vi "set Komp changes.vi"(7 "init":bool, 8 "Fehler (Eingang, kein Fehler)":errorcluster, 9 "Changes":T1, 11 "TestKonfig (Eingang) (Eingang)":T3 {"TestKonfig Interferent"."Gasflasche MFC3" items=["----"=10000, "IAG NH3 3000"=0, "IAG NH3 200"=1, "IAG NH3 2000"=2, "IAG MG"=3, "IAG O2"=4]; "TestKonfig Interferent"."Gasflasche MFC2" items=["----"=10000, "IAG NH3 3000"=0, "IAG NH3 200"=1, "IAG NH3 2000"=2, "IAG MG"=3, "IAG O2"=4]; "TestKonfig Interferent"."Eingangs Konzentration MFC1" min=0.0; "TestKonfig Interferent"."Ausgangs Konzentration MFC1" min=0.0; "TestKonfig Interferent"."MFC2" items=["MFC 2", "MFC 3", "MFC 4", "MFC 5"]; "TestKonfig Interferent"."MFC3" items=["MFC 2", "MFC 3", "MFC 4", "MFC 5"]; "TestKonfig Interferent"."Ausgangs Konzentration MFC3" min=0.0; "TestKonfig Interferent"."Eingangs Konzentration MFC3" min=0.0; "TestKonfig Interferent"."Ausgangs Konzentration MFC2" min=0.0; "TestKonfig Interferent"."Eingangs Konzentration MFC2" min=0.0; "TestKonfig H2O"."HovaCAL Temperature" format="%.2f"; "TestKonfig H2O"."HovaCAL Flow Input Cluster"."HovaCAL Flow Input Cluster" format="%.2f"; "TestKonfig H2O"."Eingangs Konzentration:" min=0.0; "TestKonfig H2O"."zusätzliche Zeitdauer Erster Punkt" min=30 step=1 format="%#_5g"; "TestKonfig H2O"."Zeitdauer Stufen" format="%#_5g"; "TestKonfig H2O"."Max Fehler" format="%#_5g"; "TestKonfig H2O"."Anzahl Stufen" format="%#_5g"; "TestKonfig H2O"."Modus" items=["Messen", "CG zu Entnahmestelle"]}) -> (0 "Fehler (Ausgang)":errorcluster, 1 "Changes  out":T1, 2 "Komponenten Name":T2, 3 "TestKonfig (Ausgang)":T3 {"TestKonfig Interferent"."Gasflasche MFC3" items=["----"=10000, "IAG NH3 3000"=0, "IAG NH3 200"=1, "IAG NH3 2000"=2, "IAG MG"=3, "IAG O2"=4]; "TestKonfig Interferent"."Gasflasche MFC2" items=["----"=10000, "IAG NH3 3000"=0, "IAG NH3 200"=1, "IAG NH3 2000"=2, "IAG MG"=3, "IAG O2"=4]; "TestKonfig Interferent"."Eingangs Konzentration MFC1" min=0.0; "TestKonfig Interferent"."Ausgangs Konzentration MFC1" min=0.0; "TestKonfig Interferent"."MFC2" items=["MFC 2", "MFC 3", "MFC 4", "MFC 5"]; "TestKonfig Interferent"."MFC3" items=["MFC 2", "MFC 3", "MFC 4", "MFC 5"]; "TestKonfig Interferent"."Ausgangs Konzentration MFC3" min=0.0; "TestKonfig Interferent"."Eingangs Konzentration MFC3" min=0.0; "TestKonfig Interferent"."Ausgangs Konzentration MFC2" min=0.0; "TestKonfig Interferent"."Eingangs Konzentration MFC2" min=0.0; "TestKonfig H2O"."HovaCAL Temperature" format="%.2f"; "TestKonfig H2O"."HovaCAL Flow Input Cluster"."HovaCAL Flow Input Cluster" format="%.2f"; "TestKonfig H2O"."Eingangs Konzentration:" min=0.0; "TestKonfig H2O"."zusätzliche Zeitdauer Erster Punkt" min=30 step=1 format="%#_5g"; "TestKonfig H2O"."Zeitdauer Stufen" format="%#_5g"; "TestKonfig H2O"."Max Fehler" format="%#_5g"; "TestKonfig H2O"."Anzahl Stufen" format="%#_5g"; "TestKonfig H2O"."Modus" items=["Messen", "CG zu Entnahmestelle"]})   [LabVIEW 2020, in "EPA 1065.lvlib" / "HovaCAL Interference verificaton.lvlib"]
uses:
  HovaCAL Interference verificaton.lvlib
  TestKonfig.ctl
  TestKonfig H2O.ctl
  Modus.ctl
  Linearisierung V2/SpanEinstellungen/Einheit.ctl
  Linearisierung V2/Gasteiler/Stufen Tabelle.ctl
  Linearisierung V2/Gasteiler/HovaCAL_Interface/Controls/Flow Einstellung.ctl
  Linearisierung V2/Gasteiler/HovaCAL_Interface/Controls/Temp Sollwerte Anzeige.ctl
  TestKonfig Interferents.ctl
  MFCAuswahl.ctl
  Seiten/System Einstellungen V2/Gasflasche Auswahl.ctl
  Visualisierungs Elemente/String - Ausgabefeld.ctl
  Konfig changes.ctl
  Aktion Index uebersetzten.ctl
  Linearisierung V2/Gasteiler/Gasteiler.lvlib
  Linearisierung V2/SpanEinstellungen/SpanEinstellungen.lvlib
  Linearisierung V2/Gasteiler/HovaCAL_Interface/Controls/Controls.lvlib
  Seiten/System Einstellungen V2/System Einstellungen V2.lvlib
panel:
  # "sec"
  # "%"
  # "sec"
  # "sec"
  # "%"
  # "sec"
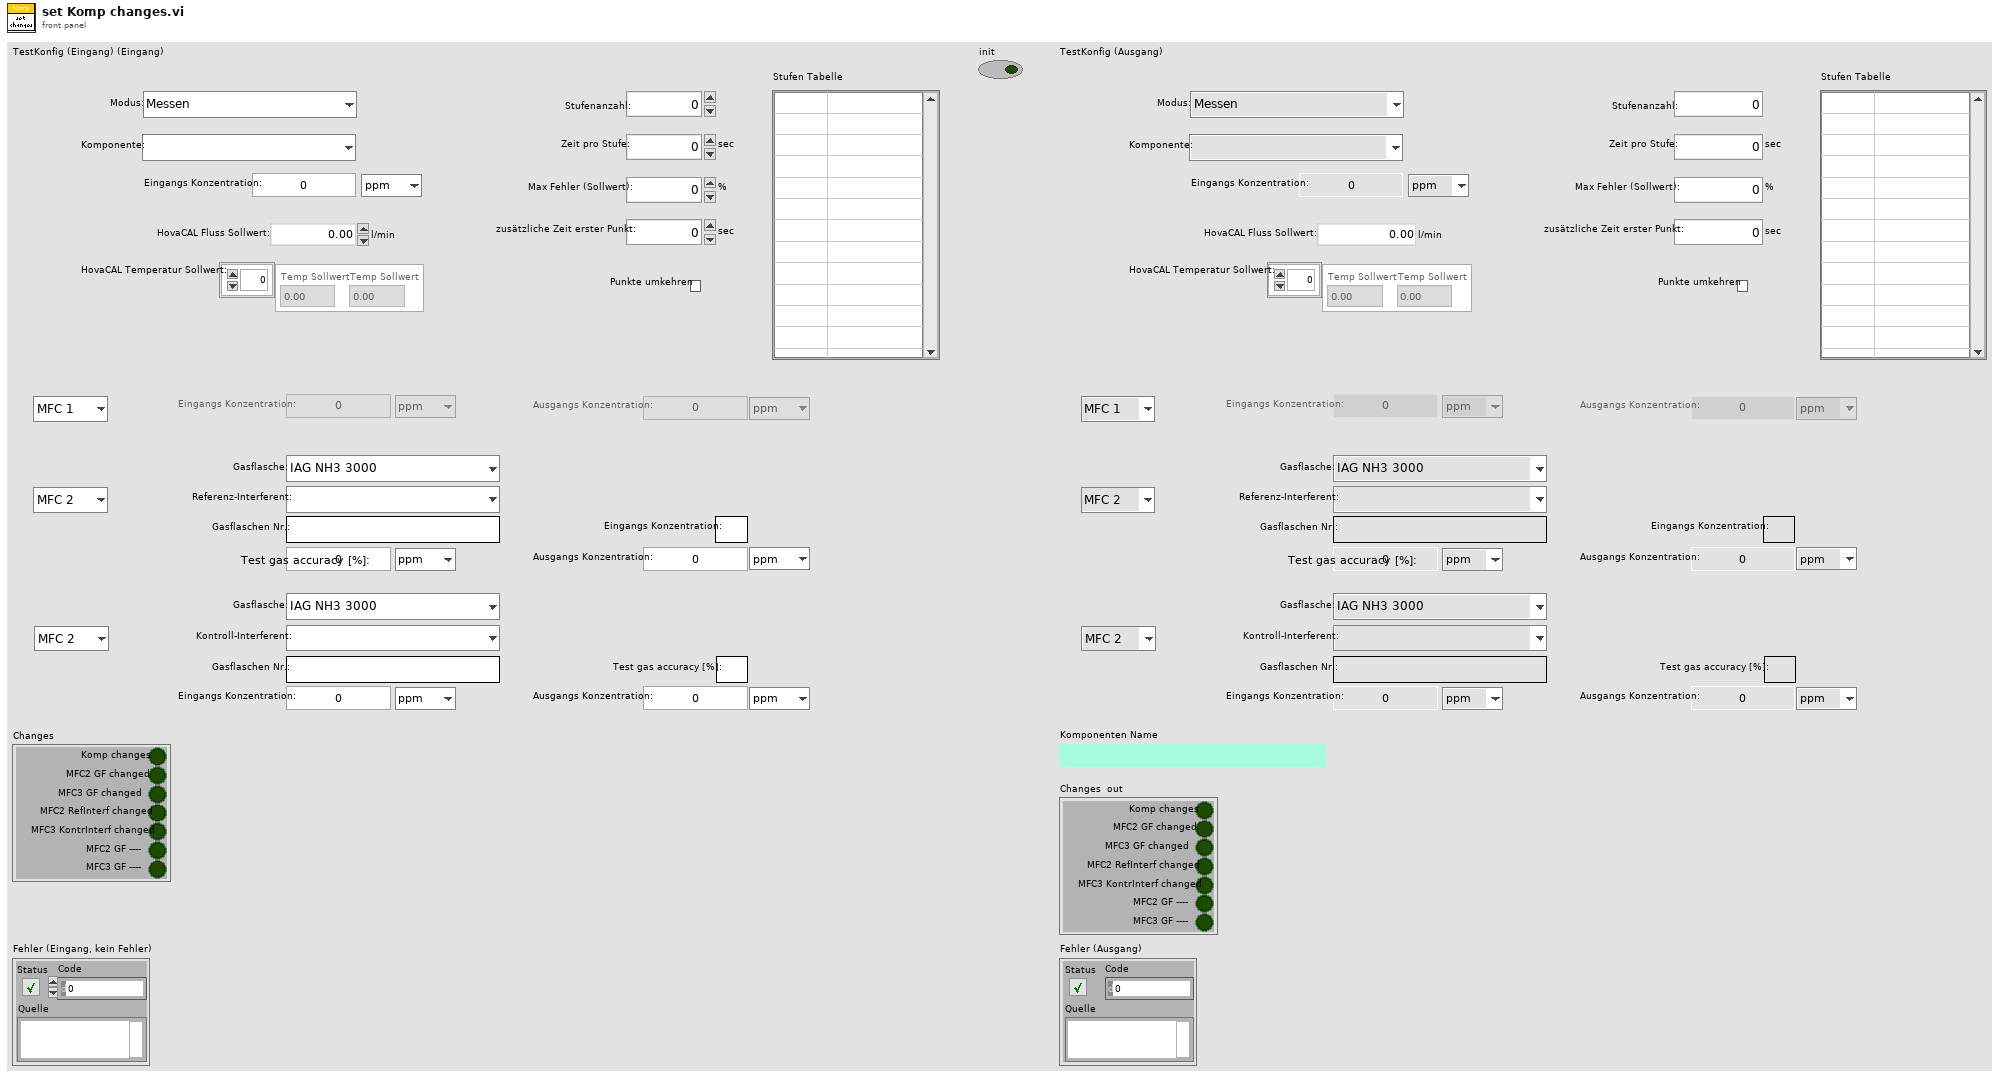
[diagram p1: front panel]
types:
  T1 = typedef "EPA 1065.lvlib/HovaCAL Interference verificaton.lvlib/Konfig changes.ctl" = cluster{"Komp changes":bool, "MFC2 GF changed":bool, "MFC3 GF changed":bool, "MFC2 RefInterf changed":bool, "MFC3 KontrInterf changed":bool, "MFC2 GF ----":bool, "MFC3 GF ----":bool}
  T2 = typedef "String - Ausgabefeld.ctl" = string
  T3 = typedef "EPA 1065.lvlib/HovaCAL Interference verificaton.lvlib/TestKonfig.ctl" = cluster{"TestKonfig H2O":T4, "TestKonfig Interferent":T10}
  T4 = typedef "EPA 1065.lvlib/HovaCAL Interference verificaton.lvlib/TestKonfig H2O.ctl" = cluster{"Modus":T5, "Komponente:":u16, "Eingangs Konzentration:":dbl, "Einheit":T6, "Anzahl Stufen":sgl, "Zeitdauer Stufen":sgl, "Max Fehler":sgl, "zusätzliche Zeitdauer Erster Punkt":sgl, "Punkte umkehren":bool, "Stufen Tabelle":T7, "HovaCAL Flow Input Cluster":T8, "HovaCAL Temperature":T9}
  T5 = typedef "EPA 1065.lvlib/HovaCAL Interference verificaton.lvlib/Modus.ctl" = u16
  T6 = typedef "Linearisierung v2.lvlib/SpanEinstellungen.lvlib/Einheit.ctl" = enum16{"ppm", "%"}
  T7 = typedef "Linearisierung v2.lvlib/Gasteiler.lvlib/Stufen Tabelle.ctl" = string[][]
  T8 = typedef "Linearisierung v2.lvlib/Gasteiler.lvlib/HovaCAL_Interface.lvlib/Controls.lvlib/Flow Einstellung.ctl" = cluster{"HovaCAL Flow Input Cluster":dbl}
  T9 = typedef "Linearisierung v2.lvlib/Gasteiler.lvlib/HovaCAL_Interface.lvlib/Controls.lvlib/Temp Sollwerte Anzeige.ctl" = dbl[]
  T10 = typedef "EPA 1065.lvlib/HovaCAL Interference verificaton.lvlib/TestKonfig Interferents.ctl" = cluster{"MFC1":enum16{"MFC 1"}, "Eingangs Konzentration MFC1":dbl, "Einheit MFC1 Eingang":T6, "Ausgangs Konzentration MFC1":dbl, "Einheit MFC1 Ausgang":T6, "MFC2":T11, "Referenz-Interferent:":u16, "Gasflaschen Nr MFC2":string, "Accuracy MFC2":string, "Eingangs Konzentration MFC2":dbl, "Einheit MFC2 Eingang":T6, "Ausgangs Konzentration MFC2":dbl, "Einheit MFC2 Ausgang":T6, "MFC3":T11, "Kontroll-Interferent:":u16, "Gasflaschen Nr MFC3":string, "Accuracy MFC3":string, "Eingangs Konzentration MFC3":dbl, "Einheit MFC3 Eingang":T6, "Ausgangs Konzentration MFC3":dbl, "Einheit MFC3 Ausgang":T6, "Gasflasche MFC2":T12, "Gasflasche MFC3":T12}
  T11 = typedef "EPA 1065.lvlib/HovaCAL Interference verificaton.lvlib/MFCAuswahl.ctl" = u16
  T12 = typedef "System Einstellungen V2.lvlib/Gasflasche Auswahl.ctl" = u16
  T13 = typedef "EPA 1065.lvlib/HovaCAL Interference verificaton.lvlib/Aktion Index uebersetzten.ctl" = enum16{"lesen", "schreiben", "auswerten", "Referenzwert", "KompIndex", "RefInterferIndex", "KontrInterfIndex"}
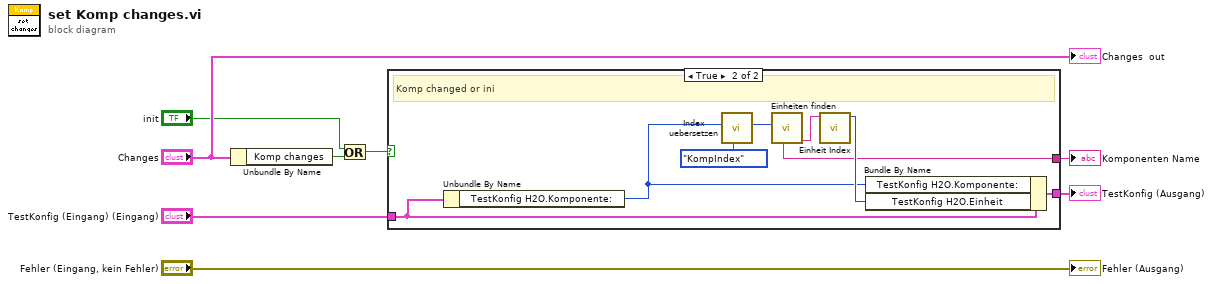
[diagram p0: block diagram]
diagram:
  n1 = Unbundle By Name("Changes") -> ("Komp changes"=w3:bool)
  n2 = Or(x="init", y=w3) -> (x .or. y?=w2:bool)
  n3 = case shown="True" w2 {
    tunnel: "TestKonfig (Eingang) (Eingang)" -> [w9 w11]
    tunnel: [w9 w17] -> w8
    tunnel: [_ w12] -> w6
    frame False {
    }
    frame True {
      # "Komp changed or ini"
      n4 = Unbundle By Name(w11) -> ("TestKonfig H2O.Komponente:"=w10:u16)
      n5 = call "Index uebersetzen.vi"("Aktion"=Aktion_Index_uebersetzten."KompIndex", "Index relativ:"=w10) -> ("Index absolut"=w13:i32)  [unwired: 4 in, 5 out]
      n6 = call "Einheiten finden.vi"("Komponente"=w13) -> ("Einheit in String"=w16:string, "Komponenten Name"=w12:T2)  [unwired: 6 in, 3 out]
      n7 = call "Einheit Index.vi"("Einheit in String"=w16) -> ("Elementindex"=w15:i32)  [unwired: 10 in]
      n8 = Bundle By Name(cluster=w11, "TestKonfig H2O.Komponente:"=w10, "TestKonfig H2O.Einheit"=w15) -> (w17:T3)
    }
  }
  "TestKonfig (Ausgang)" <- w8
  "Komponenten Name" <- w6
  "Fehler (Ausgang)" <- "Fehler (Eingang, kein Fehler)"
  "Changes  out" <- "Changes"
